vi "AVI_Test.vi"() -> ()   [LabVIEW 2009]
uses:
  <vilib>/vision/NI_Vision_Development_Module.lvlib
panel:
  out "Cores Utilized":u32
  out "Frame Duration":i64
  out "rectangle":i32[](array[numeric])=[103, 210, 569, 367]
  in  "Change ROI":bool
  out "ROI":T1(plugin-control)
  in  "Slide":u32(slide)=143 scale=0.0..3294.0
  in  "stop":bool
  out "Image":T1(plugin-control)
  out "Start Time":u32=3771410
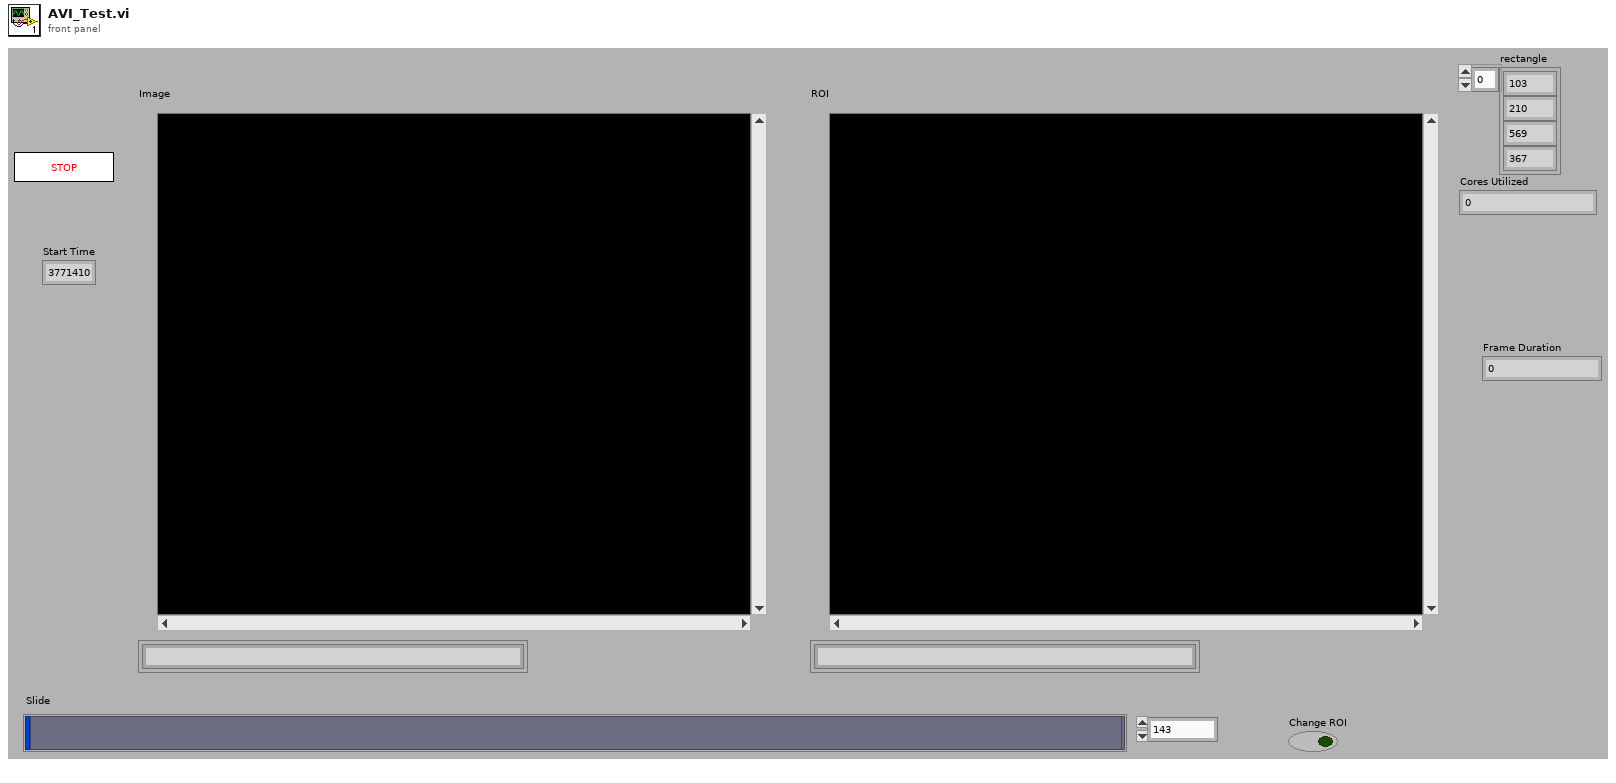
[diagram p1: front panel]
types:
  T1 = typedef "IMAQ Image.ctl" = refnum<image>
  T2 = typedef "Image Type" = u32
  T3 = enum32{"existing file", "new file", "new or existing file", "existing dir", "new dir", "new or existing dir", "existing file (use LLBs)", "new file (use LLBs)", "new or existing file (use LLBs)", "new or existing file or directory (use LLBs)"}
  T4 = typedef "AviRefnum.ctl" = refnum<k1>
  T5 = cluster{"width":u32, "height":u32, "framesPerSecond":u32, "compressionFilter":string, "hasData":bool}
  T6 = typedef "IMAQ Rectangle" = cluster{"Left":i32, "Top":i32, "Right":i32, "Bottom":i32, "Rotation":dbl}
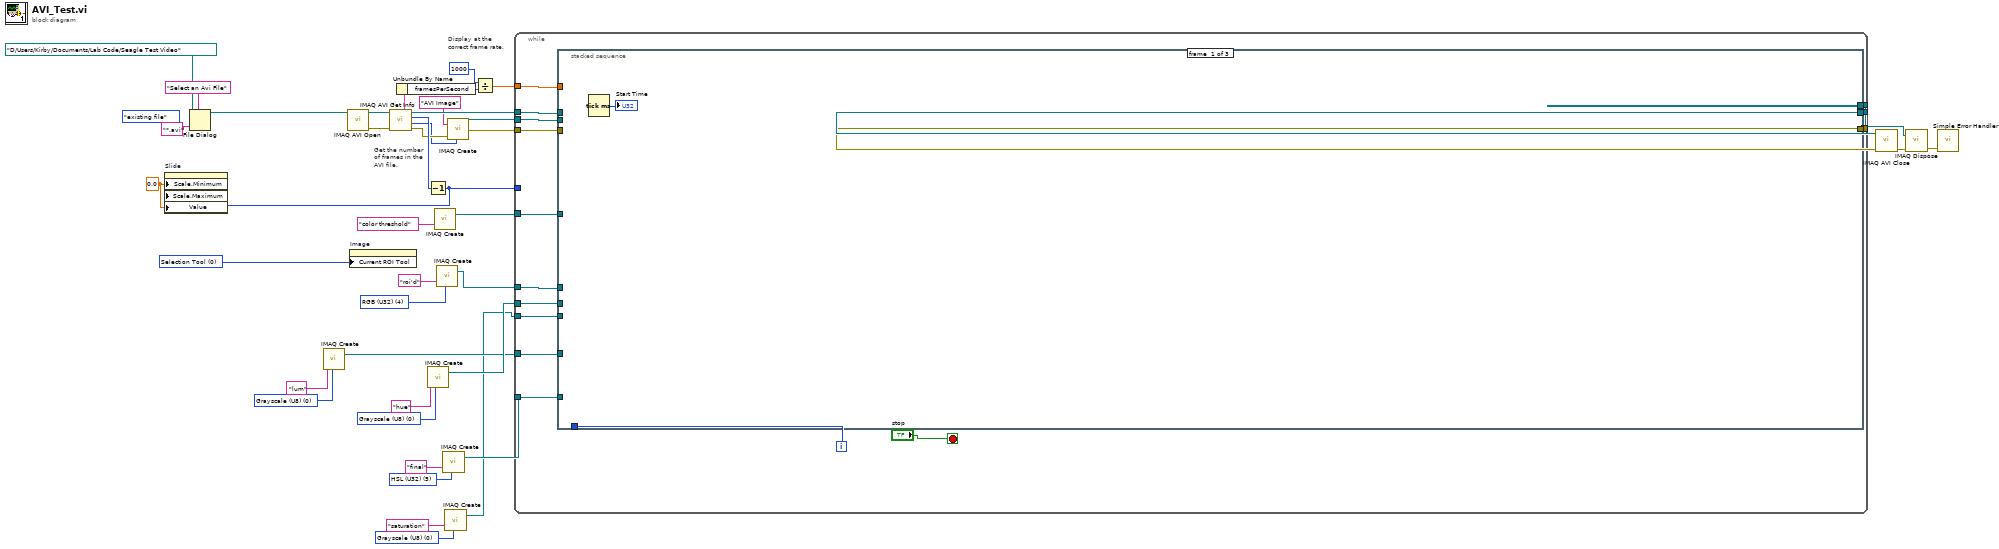
[diagram p0: block diagram]
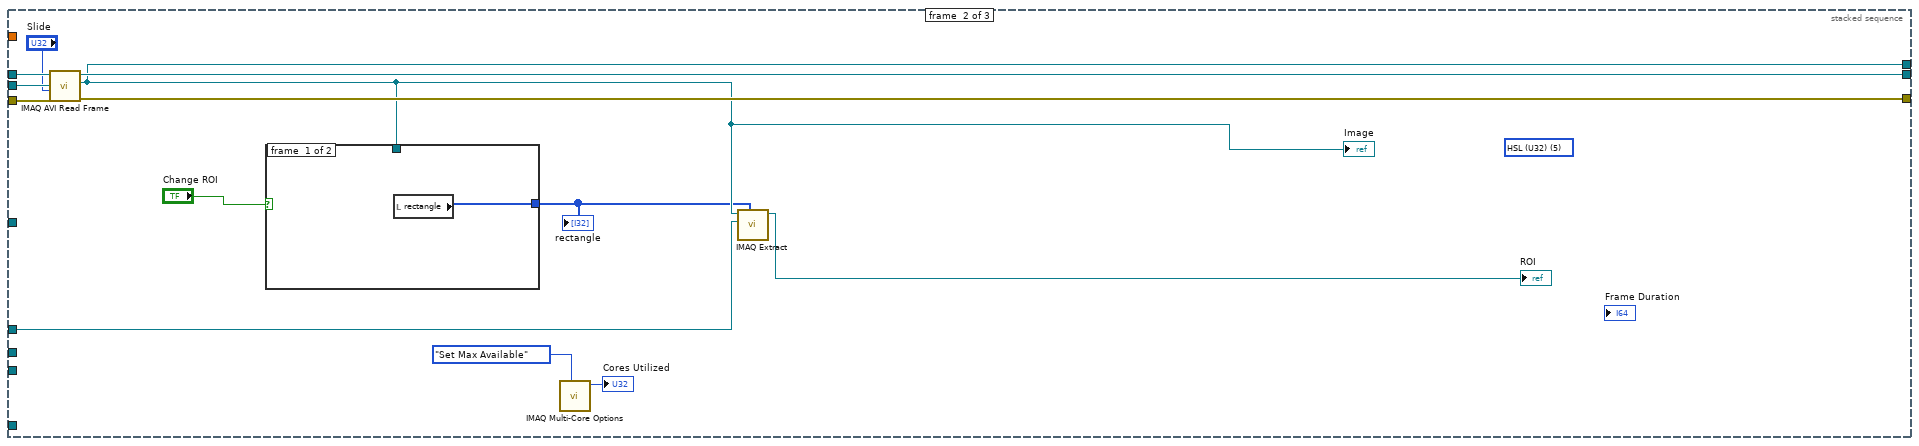
[diagram p2: hidden frame]
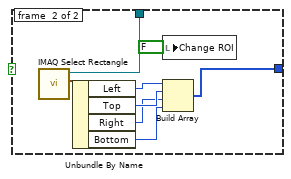
[diagram p3: hidden frame]
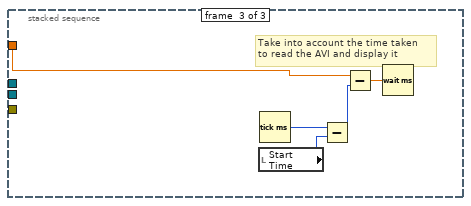
[diagram p4: hidden frame]
diagram:
  w6 = T2 0 items=["Grayscale (U8)", "Grayscale (I16)", "Grayscale (SGL)", "Complex (CSG)", "RGB (U32)", "HSL (U32)", "RGB (U64)", "Grayscale (U16)"] ("Image Type")
  w8 = T2 5 items=["Grayscale (U8)", "Grayscale (I16)", "Grayscale (SGL)", "Complex (CSG)", "RGB (U32)", "HSL (U32)", "RGB (U64)", "Grayscale (U16)"] ("Image Type")
  w10 = u32 0 items=["Zoom Tool"=8, "Selection Tool"=0, "Pan Tool"=9, "Point Tool"=1, "Line Tool"=2, "Rectangle Tool"=3, "Rotated Rectangle Tool"=12, "Polyline Tool"=10, "Polygon Tool"=5, "Freehand Tool"=11, "Closed Freehand Tool"=6, "Ellipse Tool"=4, "Annulus Tool"=7] ("Current ROI Tool")
  w2 = T2 4 items=["Grayscale (U8)", "Grayscale (I16)", "Grayscale (SGL)", "Complex (CSG)", "RGB (U32)", "HSL (U32)", "RGB (U64)", "Grayscale (U16)"] ("Image Type")
  w12 = T2 0 items=["Grayscale (U8)", "Grayscale (I16)", "Grayscale (SGL)", "Complex (CSG)", "RGB (U32)", "HSL (U32)", "RGB (U64)", "Grayscale (U16)"] ("Image Type")
  w13 = T2 0 items=["Grayscale (U8)", "Grayscale (I16)", "Grayscale (SGL)", "Complex (CSG)", "RGB (U32)", "HSL (U32)", "RGB (U64)", "Grayscale (U16)"] ("Image Type")
  w14 = 0.0 ("Scale.Range:Minimum")
  (unwired) T3."existing file" ("select mode (2)")
  # "Display at the \ncorrect frame rate."
  # "Get the number\nof frames in the\nAVI file."
  n1 = File Dialog(6:"*.avi" ("pattern"), 7:"Select an Avi File" ("prompt"), 11:path "D:/Users/Kirby/Documents/Lab Code/Seagle Test Video" ("start path")) -> (3:w23:path)  [unwired: 1 in, 6 out]
  n2 = call "IMAQ Create"("Image Name"="lum", "Image Type"=w6) -> ("New Image"=w4:T1)  [unwired: 3 in, 1 out]
  n3 = call "IMAQ AVI Open"("AVI Path"=w23) -> ("error out"=w31:errorcluster, "Avi Refnum"=w32:T4)  [unwired: 1 in, 8 out]
  n4 = property on="Image" class="ImageControl"("Current ROI Tool"=w10) -> ()  [unwired: 2 in, 2 out]
  n5 = call "IMAQ AVI Get Info"("error in (no error)"=w31, "Avi Refnum"=w32) -> ("error out"=w36:errorcluster, "Image Type"=w1:T2, "Number of Frames"=w42:u32, "Avi Refnum (duplicate)"=w39:T4, "Frame Data"=w27:T5)  [unwired: 5 out]
  n6 = Unbundle By Name(w27) -> ("framesPerSecond"=w30:u32)
  n7 = call "IMAQ Create"("Image Name"="hue", "Image Type"=w13) -> ("New Image"=w16:T1)  [unwired: 3 in, 1 out]
  n8 = Decrement(x=w42) -> (x-1=w15:u32)
  n9 = property on="Slide" class="Slide (strict)"("Scale.Minimum"=w14, "Scale.Maximum"=w15, "Value"=w14) -> ()  [unwired: 2 in, 2 out]
  n10 = call "IMAQ Create"("Image Name"="color threshold") -> ("New Image"=w21:T1)  [unwired: 4 in, 1 out]
  n11 = call "IMAQ Create"("Image Name"="roi'd", "Image Type"=w2) -> ("New Image"=w18:T1)  [unwired: 3 in, 1 out]
  n12 = call "IMAQ Create"("Image Name"="final", "Image Type"=w8) -> ("New Image"=w7:T1)  [unwired: 3 in, 1 out]
  n13 = call "IMAQ Create"("Image Name"="saturation", "Image Type"=w12) -> ("New Image"=w3:T1)  [unwired: 3 in, 1 out]
  n14 = call "IMAQ Create"("Image Name"="AVI Image", "Image Type"=w1, "error in (no error)"=w36) -> ("New Image"=w38:T1, "error out"=w37:errorcluster)  [unwired: 1 in, 1 out]
  n15 = Divide(x=1000, y=w30) -> (x/y=w29:dbl)
  n16 = while {
    tunnel: w38 -> [w54]
    tunnel: [w55] -> w34
    tunnel: [w50] -> w33
    tunnel: w29 -> [w51]
    tunnel: w37 -> [w56]
    tunnel: w39 -> [w57]
    tunnel: [w53] -> w41
    tunnel: w15 -> [_]
    tunnel: w21 -> [w49]
    tunnel: w18 -> [w48]
    tunnel: w16 -> [w47]
    tunnel: w3 -> [w46]
    tunnel: w7 -> [w44]
    tunnel: w4 -> [w43]
    i -> [w52]
    stop <- "stop" stop-if-true
    n17 = stacked-sequence {
      tunnel: w57 -> [_ w71 _]
      tunnel: w56 -> [_ w70 _]
      tunnel: [_ w69 _] -> w55
      tunnel: w54 -> [_ w68 _]
      tunnel: [_ w64 _] -> w53
      tunnel: w52 -> [_ _ _]
      tunnel: w51 -> [_ _ w81]
      tunnel: [_ w67 _] -> w50
      tunnel: w49 -> [_ _ _]
      tunnel: w48 -> [_ w62 _]
      tunnel: w47 -> [_ _ _]
      tunnel: w46 -> [_ _ _]
      tunnel: w44 -> [_ _ _]
      tunnel: w43 -> [_ _ _]
      frame #0 {
        n18 = Tick Count (ms)() -> (millisecond timer value=→"Start Time":u32)
      }
      frame #1 {
        (unwired) T2 5 items=["Grayscale (U8)", "Grayscale (I16)", "Grayscale (SGL)", "Complex (CSG)", "RGB (U32)", "HSL (U32)", "RGB (U64)", "Grayscale (U16)"] ("Image Type")
        n19 = call "IMAQ AVI Read Frame"("error in (no error)"=w70, "Frame Number"="Slide", "Image"=w68, "Avi Refnum"=w71) -> ("error out"=w67:errorcluster, "Image Out"=w64:T1, "Avi Refnum (duplicate)"=w69:T4)  [unwired: 1 in, 4 out]
        "Image" <- w64
        n20 = case shown="False" "Change ROI" {
          tunnel: w64 -> [_ w80]
          tunnel: [w72 w73] -> w63
          frame #0 {
            n21 = local read "rectangle"() -> (w72:i32[])
          }
          frame #1 {
            n22 = call "IMAQ Select Rectangle"("Image In"=w80) -> ("Rectangle"=w79:T6)  [unwired: 7 in, 3 out]
            n23 = Unbundle By Name(w79) -> ("Left"=w77:i32, "Top"=w76:i32, "Right"=w75:i32, "Bottom"=w74:i32)
            n24 = local write "Change ROI"(FALSE ("Boolean")) -> ()
            n25 = Build Array(w77, w76, w75, w74) -> (w73:i32[])
          }
        }
        "rectangle" <- w63
        n26 = call "IMAQ Multi-Core Options"("Get/Set Number of Cores (Get)"=enum32{"Get", "Set", "Set Max Available"}."Set Max Available") -> ("Cores Utilized"=→"Cores Utilized":u32)  [unwired: 9 in, 1 out]
        n27 = call "IMAQ Extract"("Optional Rectangle"=w63, "Image Dst"=w62, "Image Src"=w64) -> ("Image Dst Out"=→"ROI":T1)  [unwired: 7 in, 1 out]
      }
      frame #2 {
        # "Take into account the time taken \nto read the AVI and display it"
        n28 = local read "Start Time"() -> (w84:u32)
        n29 = Tick Count (ms)() -> (millisecond timer value=w85:u32)
        n30 = Subtract(x=w85, y=w84) -> (x-y=w83:u32)
        n31 = Subtract(x=w81, y=w83) -> (x-y=w82:dbl)
        n32 = Wait (ms)(milliseconds to wait=w82) -> ()  [unwired: 1 out]
      }
    }
  }
  n33 = call "IMAQ AVI Close"("error in (no error)"=w33, "Avi Refnum"=w34) -> ("error out"=w40:errorcluster)  [unwired: 9 out]
  n34 = call "IMAQ Dispose"("Image"=w41, "error in (no error)"=w40) -> ("error out"=w26:errorcluster)  [unwired: 1 in, 3 out]
  n35 = call <vilib>:"Simple Error Handler.vi"("error in (no error)"=w26) -> ()  [unwired: 1 in, 8 out]
